vi "Analog Output (Host).vi"() -> ()   [LabVIEW 2011]
doc: "This VI will will initialize the FPGA VI and then continually write single point values to 4 channels of an analog output module."
uses:
  <vilib>/rvi/interface/nirviReadWriteControl/nirviReadWriteControl.xnode
  <vilib>/rvi/interface/nirviCloseFPGA/nirviCloseFPGA.xnode
  <vilib>/rvi/interface/nirviOpenFPGA/nirviOpenFPGA.xnode
  Analog Output (FPGA).vi
  FPGA Bitfiles/MAXCATTestProjec_FPGATarget3_AnalogOutput(FPG_E757C5F4.lvbitx
panel:
  in  "AO3 (V)":dbl(slide)=1.0 caption="Analog  Output AO3" scale=-10.0..10.0 scale format="%.3f"
  in  "AO2 (V)":dbl(slide)=1.0 caption="Analog Output AO2" scale=-10.0..10.0 scale format="%.3f"
  in  "AO1 (V)":dbl(slide)=1.0 caption="Analog Output AO1" scale=-10.0..10.0 scale format="%.3f"
  in  "AO0 (V)":dbl(slide)=1.0 caption="Analog Output AO0" scale=-10.0..10.0 scale format="%.3f"
  in  "Software Loop Time (ms)":u32=100
  in  "stop":bool
  # "For instructions, select Help>>Show Context Help"
  # "Resource Parameters"
  # "Timing Parameters"
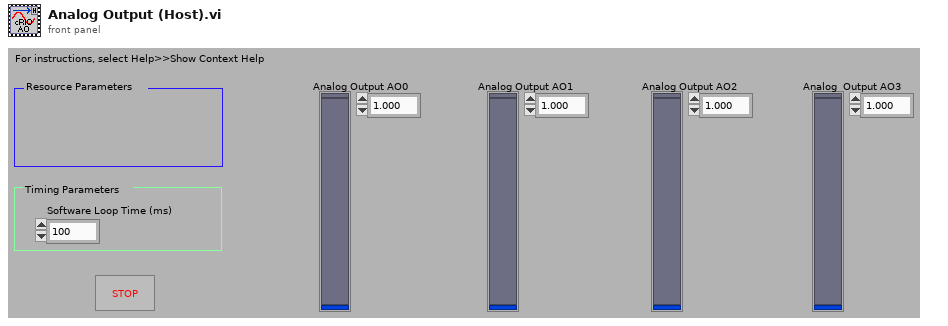
[diagram p1: front panel]
types:
  T1 = cluster{"[0]":dbl, "[1]":dbl, "[2]":dbl, "[3]":dbl}
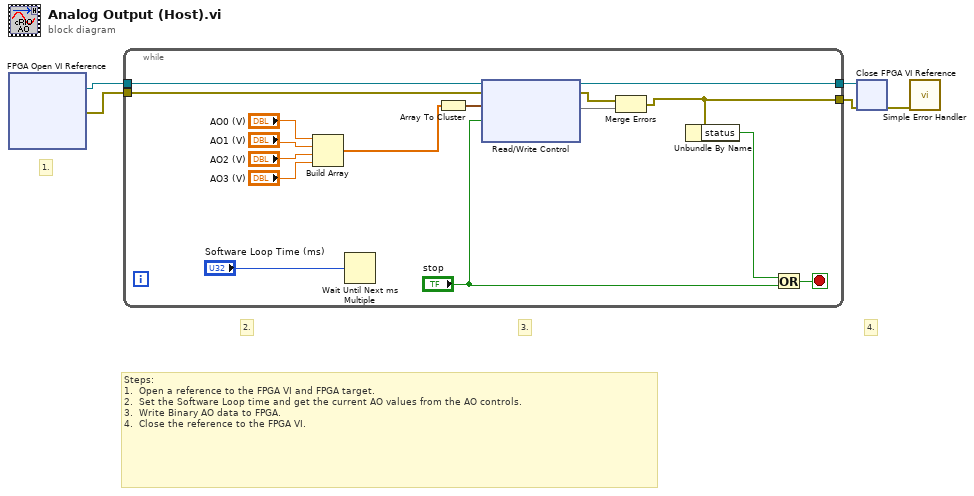
[diagram p0: block diagram]
diagram:
  # "3."
  # "4."
  # "2."
  # "1."
  # "Steps: \n1.  Open a reference to the FPGA VI and FPGA target.\n2.  Set the Software Loop time and get the current AO values from the AO controls. \n3.  Write Binary AO data to FPGA.\n4.  Close the reference to the FPGA VI."
  n1 = xnode "FPGA Open VI Reference"() -> ("FPGA VI Reference Out"=w2:refnum<k20>, "error out"=w1:errorcluster)  [unwired: 2 in]
  n2 = while {
    tunnel: w2 -> [w20]
    tunnel: [w21] -> w5
    tunnel: w1 -> [w18]
    tunnel: [w11] -> w4
    stop <- w15 stop-if-true
    n3 = Build Array("AO0 (V)", "AO1 (V)", "AO2 (V)", "AO3 (V)") -> (w6:dbl[])
    n4 = Wait Until Next ms Multiple(millisecond multiple="Software Loop Time (ms)") -> ()  [unwired: 1 out]
    n5 = Array To Cluster(array=w6) -> (cluster=w19:T1)
    n6 = xnode "Read/Write Control"("FPGA VI Reference In"=w20, "error in"=w18, "AO Data"=w19, "stop"="stop") -> ("FPGA VI Reference Out"=w21:refnum<k20>, "error out"=w13:errorcluster, "FPGA Error Out"=w12)
    n7 = Merge Errors(w13, w12) -> (w11:errorcluster)
    n8 = Unbundle By Name(w11) -> ("status"=w17:bool)
    n9 = Or(x=w17, y="stop") -> (x .or. y?=w15:bool)
  }
  n10 = xnode "Close FPGA VI Reference"("FPGA VI Reference In"=w5, "error in"=w4) -> ("error out"=w3:errorcluster)
  n11 = call <vilib>:"Simple Error Handler.vi"("error in (no error)"=w3) -> ()  [unwired: 1 in, 8 out]
